vi "Install Package.vi"(8 "error in (no error)":errorcluster, 11 "Package in":refnum<class "Package.lvclass">) -> (0 "error out":errorcluster, 3 "Package out":refnum<class "Package.lvclass">)   [LabVIEW 2020, in "neg-pkg.lvlib" / "Package.lvclass"]
uses:
  Package.lvclass
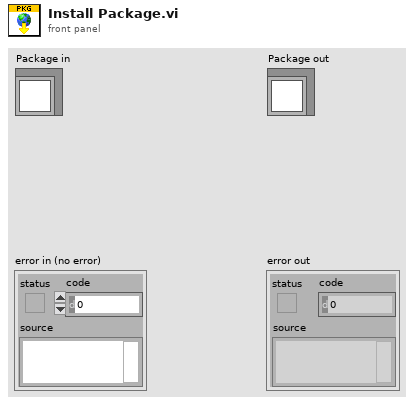
[diagram p1: front panel]
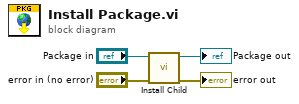
[diagram p0: block diagram]
diagram:
  n1 = call-dynamic "Install Child.vi"("error in (no error)"="error in (no error)", "Package in"="Package in") -> ("error out"=→"error out":errorcluster, "Package out"=→"Package out":refnum<class "Package.lvclass">)  [unwired: 8 in]
